vi "SelectSerialPort.vi"(8 "Error In":errorcluster) -> (0 "Error Out":errorcluster, 3 "MotorController out":refnum<class "MotorController.lvclass">)   [LabVIEW 2019]
doc: "Select the appropriate serial port."
uses:
  MotorController.lvclass
  SelectSerialPort_states_enum_typedef.ctl
  enable_disable_enum_typedef.ctl
panel:
  in  "Port":refnum<visa-resource-name>
  in  "Next":bool
  # "Motor Controller Port"
  # "Select the correct serial port for the motor controller. Motors will be\nconnected to and enabled."
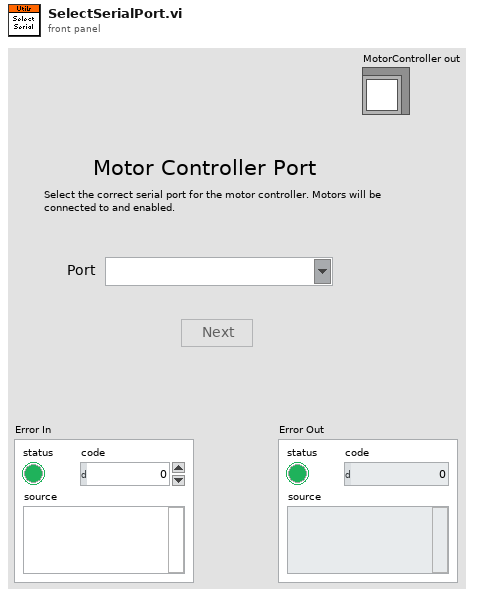
[diagram p1: front panel]
types:
  T1 = typedef "SelectSerialPort_states_enum_typedef.ctl" = enum16{"Shutdown", "Connect", "Wait", "Initialize"}
  T2 = enum8{"Enabled", "Disabled", "Disabled and Grayed Out"}
  T3 = typedef "MotorController.lvclass/enable_disable_enum_typedef.ctl" = enum16{"Enable", "Disable"}
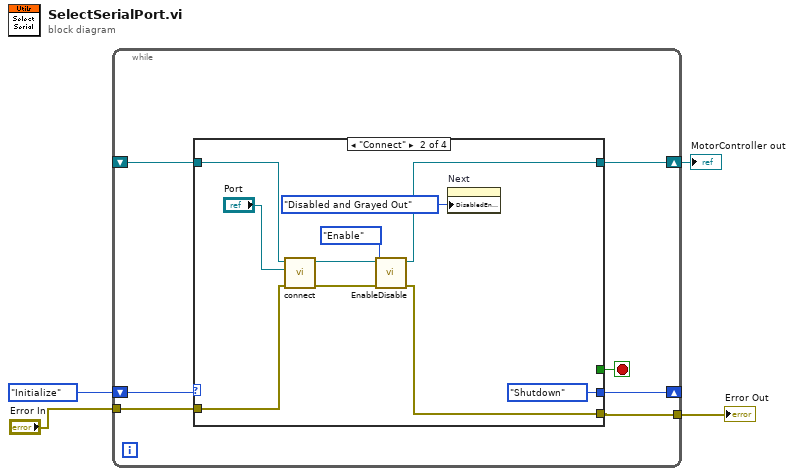
[diagram p0: block diagram]
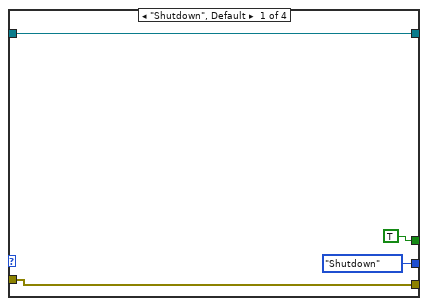
[diagram p2: hidden frame]
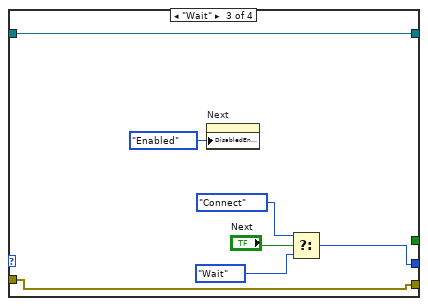
[diagram p3: hidden frame]
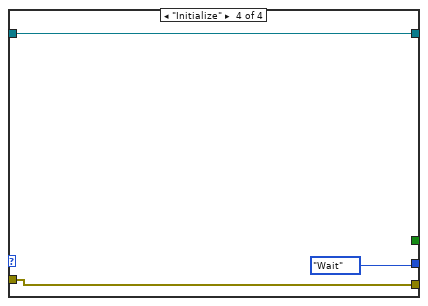
[diagram p4: hidden frame]
diagram:
  n1 = while {
    shift-right: [w8] -> _
    shift-left: SelectSerialPort_states_enum_typedef."Initialize" -> [w11]
    tunnel: "Error In" -> [w10]
    tunnel: [w9] -> w2
    shift-right: [w7] -> w1
    shift-left: _ -> [w6]
    stop <- w5 stop-if-true
    n2 = case shown="\"Connect\"" w11 {
      tunnel: w10 -> [w13 w22 w28 w35]
      tunnel: [w13 w18 w28 w35] -> w9
      tunnel: [SelectSerialPort_states_enum_typedef."Shutdown" SelectSerialPort_states_enum_typedef."Shutdown" w29 SelectSerialPort_states_enum_typedef."Wait"] -> w8
      tunnel: [w15 w20 w27 w33] -> w7
      tunnel: w6 -> [w15 w19 w27 w33]
      tunnel: [TRUE _ _ _] -> w5
      frame "Shutdown", Default {
      }
      frame "Connect" {
        n3 = call "connect.vi"("error in (no error)"=w22, "Serial Port"="Port", "MotorController in"=w19) -> ("error out"=w24:errorcluster, "MotorController out"=w25:refnum<class "MotorController.lvclass">)  [unwired: 7 in]
        n4 = call "EnableDisable.vi"("error in (no error)"=w24, "Action"=enable_disable_enum_typedef."Enable", "MotorController in"=w25) -> ("error out"=w18:errorcluster, "MotorController out"=w20:refnum<class "MotorController.lvclass">)  [unwired: 7 in]
        n5 = property on="Next" class="Bool"("DisabledEnum"=T2."Disabled and Grayed Out" ("Disabled")) -> ()  [unwired: 2 in, 2 out]
      }
      frame "Wait" {
        n6 = property on="Next" class="Bool"("DisabledEnum"=T2."Enabled" ("Disabled")) -> ()  [unwired: 2 in, 2 out]
        n7 = Select(t=SelectSerialPort_states_enum_typedef."Connect", s="Next", f=SelectSerialPort_states_enum_typedef."Wait") -> (s? t:f=w29:T1)
      }
      frame "Initialize" {
      }
    }
  }
  "Error Out" <- w2
  "MotorController out" <- w1
